vi "CRYFlatten Windows System.vi"(11 "Windows System":T1) -> (3 "WinSys flattened":string)   [LabVIEW 2013]
uses:
  Control/CRYWindows Sysem.ctl
  <vilib>/Utility/miscctls.llb/LVRectTypeDef.ctl
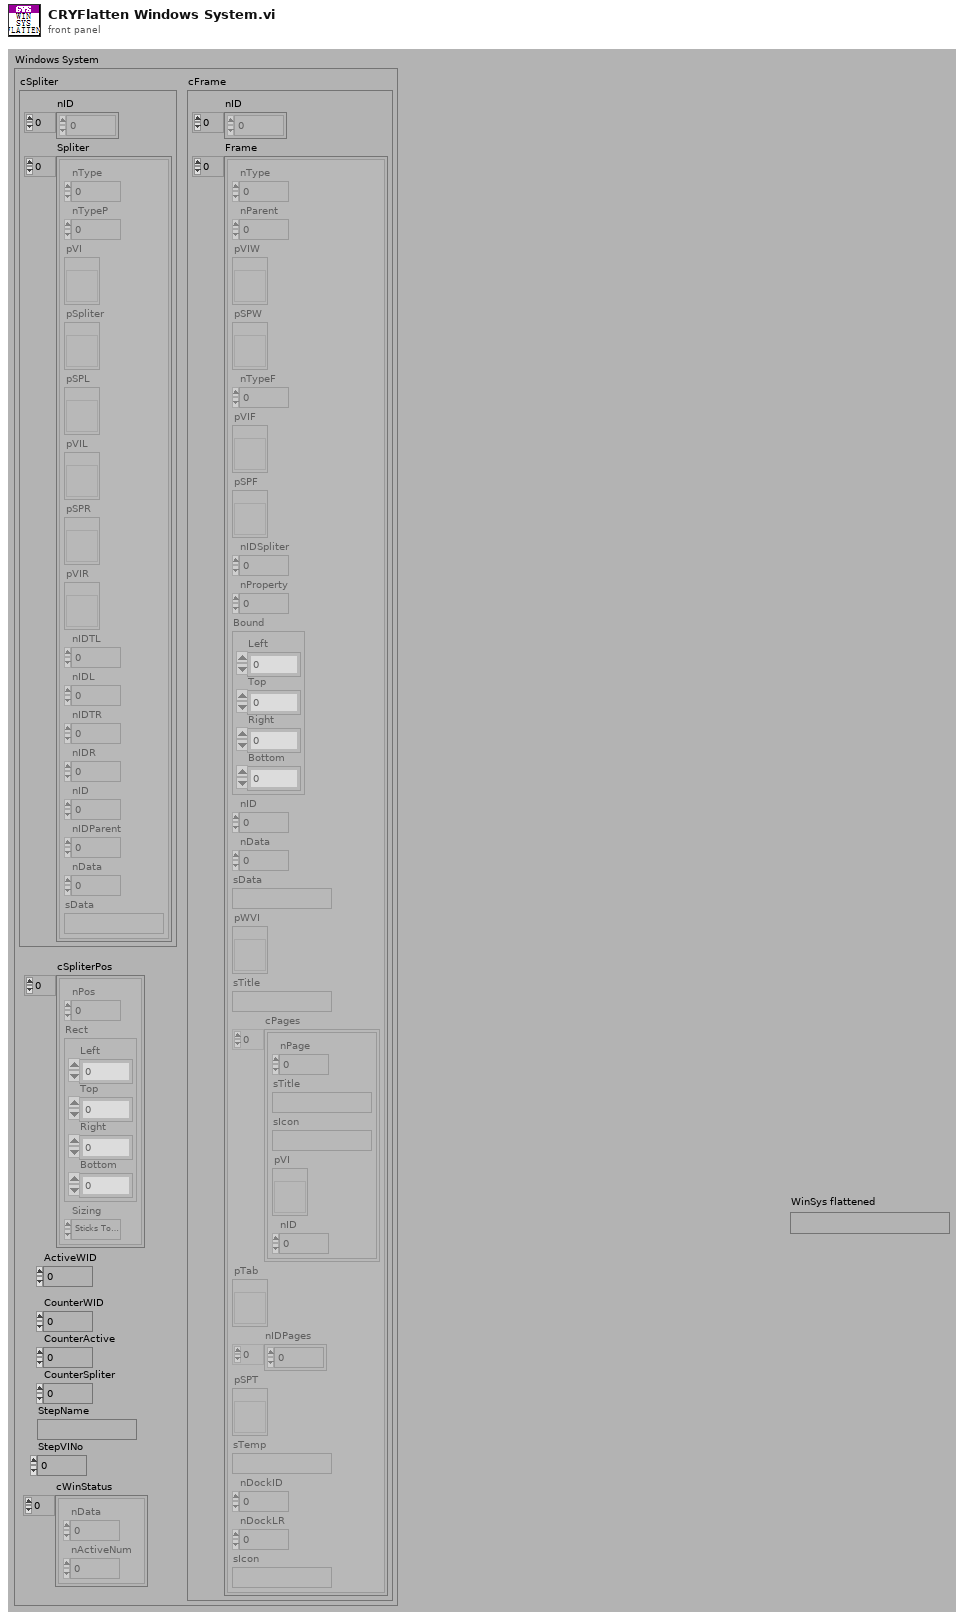
[diagram p1: front panel]
types:
  T1 = typedef "CRYWindows Sysem.ctl" = cluster{"cFrame":cluster{"nID":i32[], "Frame":cluster{"nType":i32, "nParent":i32, "pVIW":refnum<vi>, "pSPW":refnum<vi>, "nTypeF":i32, "pVIF":refnum<vi>, "pSPF":refnum<vi>, "nIDSpliter":i32, "nProperty":i32, "Bound":T2, "nID":i32, "nData":i32, "sData":string, "pWVI":refnum<vi>, "sTitle":string, "cPages":cluster{"nPage":i32, "sTitle":string, "sIcon":string, "pVI":refnum<vi>, "nID":i32}[], "pTab":refnum<vi>, "nIDPages":i32[], "pSPT":refnum<vi>, "sTemp":string, "nDockID":i32, "nDockLR":i32, "sIcon":string}[]}, "cSpliter":cluster{"nID":i32[], "Spliter":cluster{"nType":i32, "nTypeP":i32, "pVI":refnum<vi>, "pSpliter":refnum<vi>, "pSPL":refnum<vi>, "pVIL":refnum<vi>, "pSPR":refnum<vi>, "pVIR":refnum<vi>, "nIDTL":i32, "nIDL":i32, "nIDTR":i32, "nIDR":i32, "nID":i32, "nIDParent":i32, "nData":i32, "sData":string}[]}, "ActiveWID":i32, "cSpliterPos":cluster{"nPos":i32, "Rect":T2, "Sizing":enum16{"Sticks Top/Left", "Sticks Bottom/Right", "Proportional"}}[], "CounterWID":i32, "CounterActive":i32, "CounterSpliter":i32, "cWinStatus":cluster{"nData":i32, "nActiveNum":i32}[], "StepName":string, "StepVINo":i32}
  T2 = typedef "LVRectTypeDef.ctl" = cluster{"Left":i16, "Top":i16, "Right":i16, "Bottom":i16}
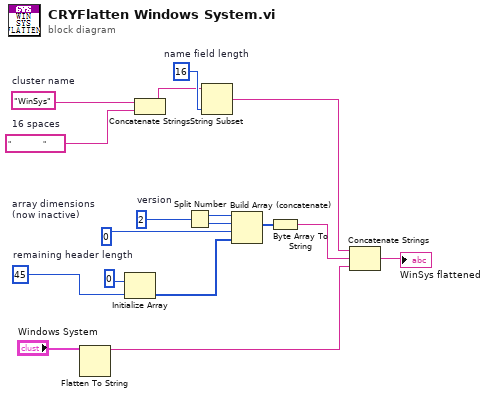
[diagram p0: block diagram]
diagram:
  w3 = u8 0  # array dimensions (now inactive)
  w6 = 16  # name field length
  w7 = "                "  # 16 spaces
  w8 = "WinSys"  # cluster name
  w13 = 45  # remaining header length
  w17 = u16 2  # version
  n1 = Flatten To String(anything="Windows System") -> (data string=w2:string)  [unwired: 1 in, 4 out]
  n2 = Initialize Array(u8 0, w13) -> (w9:u8[])
  n3 = Concatenate Strings(w8, w7) -> (w5:string)
  n4 = Split Number(x=w17) -> (hi(x)=w16:u8, lo(x)=w15:u8)
  n5 = String Subset(string=w5, length (rest)=w6) -> (substring=w4:string)  [unwired: 1 out]
  n6 = Build Array (concatenate)(w16, w15, w3, w9) -> (w12:u8[])
  n7 = Byte Array To String(unsigned byte array=w12) -> (string=w10:string)
  n8 = Concatenate Strings(w4, w10, w2) -> (→"WinSys flattened":string)
